vi "WriteOutput.vi"(5 "Output type":i16, 6 "Number of Samples":i32, 7 "Output FIFO":refnum<k21>, 9 "Average":sgl[](array[numeric])=[0.0, 0.0, 0.0, 0.0, 0.0, 0.0, 0.0, 0.0, 0.0], 10 "Max":fxp<+/-,24,4>[](array[numeric])=[0.0, 0.0, 0.0, 0.0, 0.0, 0.0, 0.0, 0.0, 0.0], 11 "Min":fxp<+/-,24,4>[](array[numeric])=[0.0, 0.0, 0.0, 0.0, 0.0, 0.0, 0.0, 0.0, 0.0]) -> (3 "FIFO full":bool)   [LabVIEW 2018]
uses:
  <vilib>/rvi/DataTransferAndStorage/Container/Common/niFpgaContainerExecOnDevCompGetState.vi
  <vilib>/rvi/Emulation/niFpgaEmulationIsFPGAContextNoSignature.vi
  <vilib>/rvi/Emulation/niFpgaSctlEmulationGetInTimedLoop.vi
  <vilib>/rvi/errors/niFpgaSetErrorForExecOnDevCompSimple.vi
  <vilib>/rvi/eio/common/nirviEmuReportErrorAndStop.vi
  <vilib>/rvi/DataTransferAndStorage/Container/Common/niFpgaContainerGetUniqueNameForEmu.vi
  <vilib>/rvi/FIFO/Fifo_Resource/nirvififoEmulationSetSize.vi
  <vilib>/rvi/FIFO/Fifo_Resource/nirviFifoEmulationQueueMgr.vi
  <instcachedir>/0/nirviFifoEmulationQueueMgr_E5CAEC123FF24DC58D834DCA3CDAA9B5.lvgen/nirviFifoEmulationQueueMgr_E5CAEC123FF24DC58D834DCA3CDAA9B5_004.vi
  <vilib>/rvi/FIFO/Fifo_Resource/nirvififoEmulationDetermineInputValidOut.vi
  <vilib>/rvi/FIFO/Fifo_Resource/nirvififoEmulationCreateLock.vi
  <vilib>/rvi/Emulation/niFpgaProcessEmulError.vi
  <vilib>/rvi/FIFO/Fifo_Resource/nirvififoEmulationObtainLock.vi
  <vilib>/rvi/FIFO/Fifo_Resource/nirvififoEmulationReleaseLock.vi
  <vilib>/rvi/occurrence/nirviWaitOnOccurrenceBase.vi
  <vilib>/rvi/errors/nirviReportUnexpectedCaseInternalError.vi
  <vilib>/rvi/errors/nirviReportUnexpectedCaseInternalError (U32).vi
  <vilib>/Utility/error.llb/Clear Errors.vi
  <vilib>/rvi/interface/RandomDataEmulation/niFpgaRandomDataHandleErrors.vi
  <vilib>/rvi/DataTransferAndStorage/Container/XNode/niFpgaContainer.xnode
  <vilib>/rvi/FIFO/Fifo_Resource/niFpgaFifoEmulationRefIn.vi
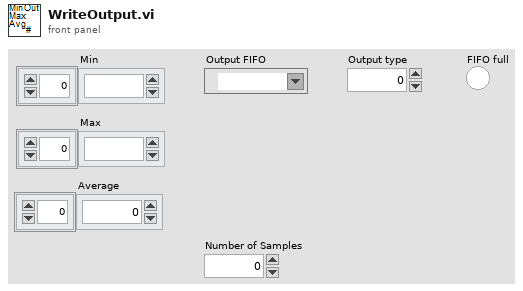
[diagram p1: front panel]
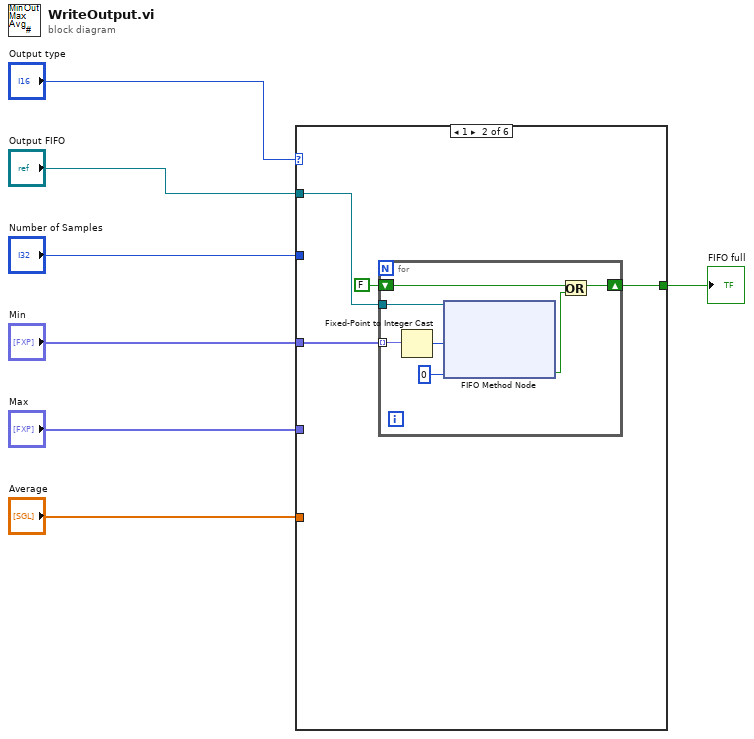
[diagram p0: block diagram]
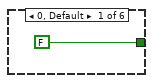
[diagram p2: hidden frame]
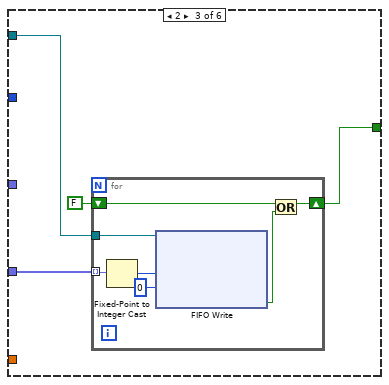
[diagram p3: hidden frame]
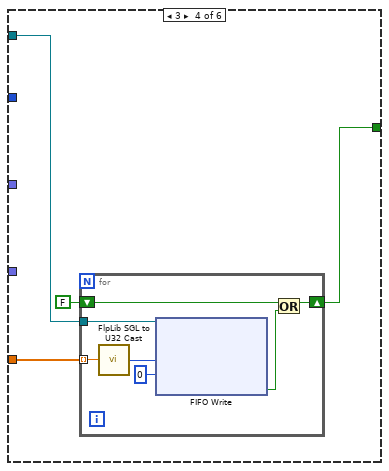
[diagram p4: hidden frame]
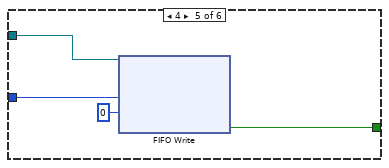
[diagram p5: hidden frame]
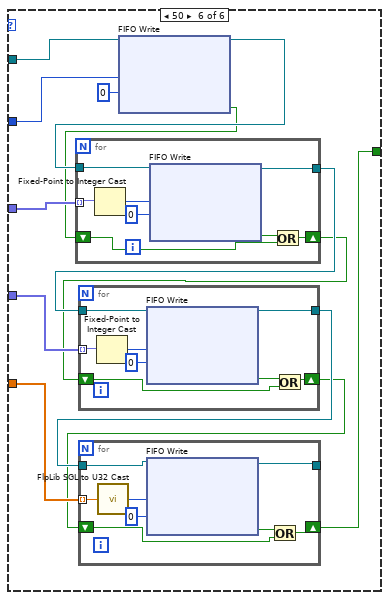
[diagram p6: hidden frame]
diagram:
  n1 = case shown="1" "Output type" {
    tunnel: "Output FIFO" -> [_ w12 w23 w34 w45 w53]
    tunnel: "Min" -> [_ w11 _ _ _ w58]
    tunnel: "Max" -> [_ _ w22 _ _ w56]
    tunnel: "Average" -> [_ _ _ w33 _ w54]
    tunnel: "Number of Samples" -> [_ _ _ _ w44 w51]
    tunnel: [FALSE ("Timed Out?") w10 w21 w32 w42 w49] -> w1
    frame 0, Default {
    }
    frame 1 {
      n2 = for {
        tunnel: w12 -> [w19]
        tunnel: w11 -> [w18] mode=indexing
        shift-right: [w16] -> w10
        shift-left: FALSE ("Timed Out?") -> [w15]
        n3 = Fixed-Point to Integer Cast(1:w18) -> (0:w13:i32)
        n4 = xnode ("FIFO Method Node")("Element"=w13, "Timeout"=0, "FIFO In"=w19) -> ("Timed Out?"=w14:bool)  [unwired: 1 out]
        n5 = Or(x=w15, y=w14) -> (x .or. y?=w16:bool)
      }
    }
    frame 2 {
      n6 = for {
        tunnel: w23 -> [w30]
        tunnel: w22 -> [w28] mode=indexing
        shift-right: [w27] -> w21
        shift-left: FALSE -> [w25]
        n7 = Fixed-Point to Integer Cast(1:w28) -> (0:w24:i32)
        n8 = xnode ("FIFO Write")("Element"=w24, "Timeout"=0, "FIFO In"=w30) -> ("Timed Out?"=w26:bool)  [unwired: 1 out]
        n9 = Or(x=w25, y=w26) -> (x .or. y?=w27:bool)
      }
    }
    frame 3 {
      n10 = for {
        tunnel: w34 -> [w41]
        tunnel: w33 -> [w36] mode=indexing
        shift-right: [w39] -> w32
        shift-left: FALSE ("Timed Out?") -> [w37]
        n11 = call <userlib>:"FlpLib SGL to U32 Cast.vi"("x"=w36) -> ("y"=w35:u32)  [unwired: 4 in]
        n12 = xnode ("FIFO Write")("Element"=w35, "Timeout"=0, "FIFO In"=w41) -> ("Timed Out?"=w38:bool)  [unwired: 1 out]
        n13 = Or(x=w37, y=w38) -> (x .or. y?=w39:bool)
      }
    }
    frame 4 {
      n14 = xnode ("FIFO Write")("Element"=w44, "Timeout"=0, "FIFO In"=w45) -> ("Timed Out?"=w42:bool)  [unwired: 1 out]
    }
    frame 50 {
      n15 = xnode ("FIFO Write")("Element"=w51, "Timeout"=0, "FIFO In"=w53) -> ("Timed Out?"=w46:bool, "FIFO Out"=w52:refnum<k21>)
      n16 = for {
        tunnel: w52 -> [w82]
        tunnel: w58 -> [w81] mode=indexing
        tunnel: [w79] -> w57
        shift-right: [w78] -> w47
        shift-left: w46 -> [w76]
        n17 = Fixed-Point to Integer Cast(1:w81) -> (0:w75:i32)
        n18 = xnode ("FIFO Write")("Element"=w75, "Timeout"=0, "FIFO In"=w82) -> ("Timed Out?"=w77:bool, "FIFO Out"=w79:refnum<k21>)
        n19 = Or(x=w77, y=w76) -> (x .or. y?=w78:bool)
      }
      n20 = for {
        tunnel: w57 -> [w74]
        tunnel: w56 -> [w73] mode=indexing
        tunnel: [w71] -> w55
        shift-right: [w69] -> w48
        shift-left: w47 -> [w68]
        n21 = Fixed-Point to Integer Cast(1:w73) -> (0:w67:i32)
        n22 = xnode ("FIFO Write")("Element"=w67, "Timeout"=0, "FIFO In"=w74) -> ("Timed Out?"=w70:bool, "FIFO Out"=w71:refnum<k21>)
        n23 = Or(x=w70, y=w68) -> (x .or. y?=w69:bool)
      }
      n24 = for {
        tunnel: w55 -> [w66]
        tunnel: w54 -> [w60] mode=indexing
        tunnel: [w64] -> _
        shift-right: [w63] -> w49
        shift-left: w48 -> [w61]
        n25 = call <userlib>:"FlpLib SGL to U32 Cast.vi"("x"=w60) -> ("y"=w59:u32)  [unwired: 4 in]
        n26 = xnode ("FIFO Write")("Element"=w59, "Timeout"=0, "FIFO In"=w66) -> ("Timed Out?"=w62:bool, "FIFO Out"=w64:refnum<k21>)
        n27 = Or(x=w62, y=w61) -> (x .or. y?=w63:bool)
      }
    }
  }
  "FIFO full" <- w1
